vi "Launcher.vi"() -> ()   [LabVIEW 2021]
uses:
  <vilib>/ActorFramework/Actor/Actor.lvclass
  Async Methods Actor Example.lvclass
  C:/Projects/Async Actors/Async Actor/Async Methods Actor/Async Methods Actor.lvclass
  C:/Program Files/National Instruments/LabVIEW 2021/vi.lib/ActorFramework/Actor/Actor.lvclass
  C:/Projects/Async Actors/Async Actor Example/Async Actor Example/Async Methods Actor Example.lvclass
panel:
  out "error out":errorcluster
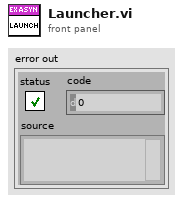
[diagram p1: front panel]
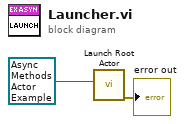
[diagram p0: block diagram]
diagram:
  n1 = call <vilib>:"Launch Root Actor.vi"("Actor"=refnum<class "Async Methods Actor Example.lvclass"> refnum ("Async Actor Example.lvlib:Async Actor Example.lvclass")) -> ("error out"=→"error out":errorcluster)  [unwired: 9 in, 1 out]
